vi "Part 1.vi"(11 "Input":string) -> (3 "Output":i64)   [LabVIEW 2021]
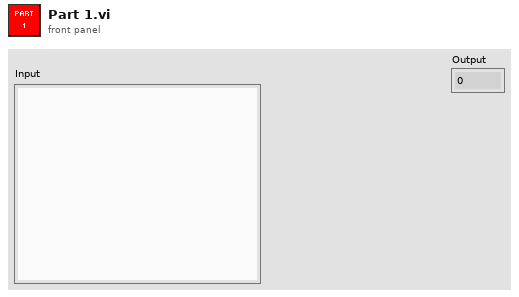
[diagram p1: front panel]
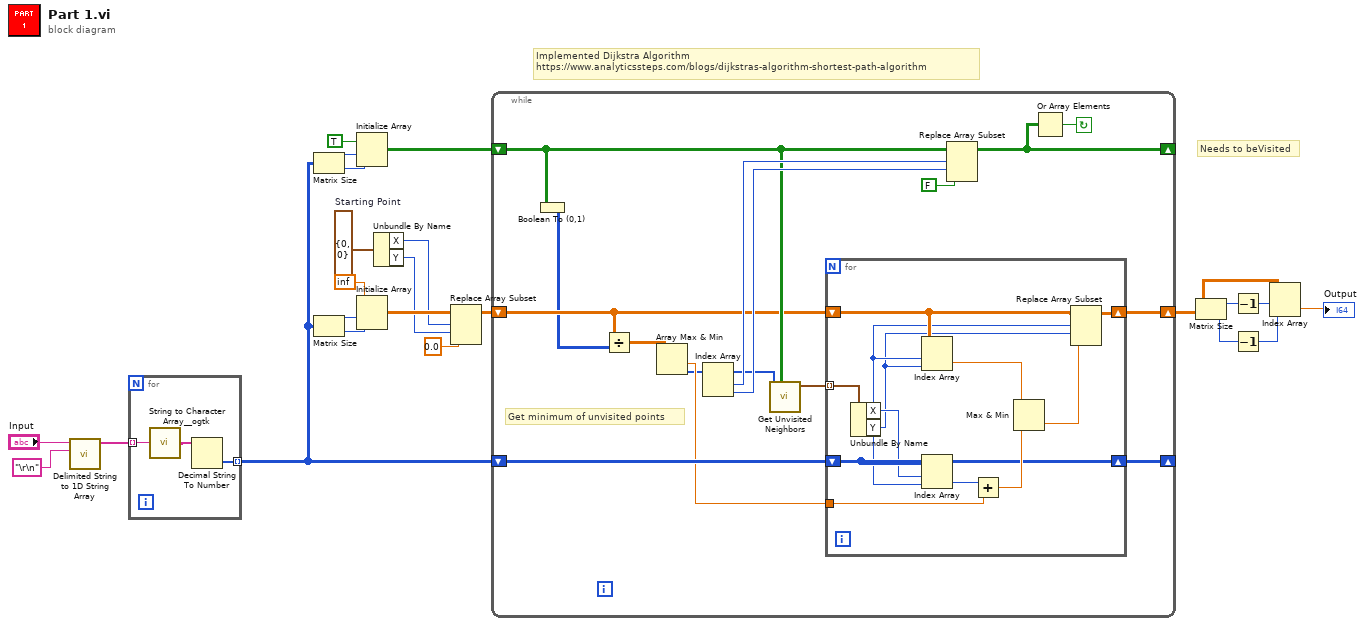
[diagram p0: block diagram]
diagram:
  w9 = cluster{"X":i32, "Y":i32} {"X"=0, "Y"=0}  # Starting Point
  # "Implemented Dijkstra Algorithm\nhttps://www.analyticssteps.com/blogs/dijkstras-algorithm-shortest-path-algorithm"
  # "Needs to beVisited"
  n1 = call <vilib>:"Delimited String to 1D String Array.vi"("delimiter"="\r\n", "delimited string"="Input") -> ("string array"=w21:string[])  [unwired: 9 in]
  n2 = for {
    tunnel: w21 -> [w26] mode=indexing
    tunnel: [w24] -> w12 mode=indexing
    n3 = call <userlib>:"String to Character Array__ogtk.vi"("Input String"=w26) -> ("Character Array"=w25:string[])
    n4 = Decimal String To Number(string=w25) -> (number=w24:i32[])  [unwired: 2 in, 1 out]
  }
  n5 = Matrix Size(0:w12) -> (1:w20:i32, 2:w19:i32)
  n6 = Matrix Size(0:w12) -> (1:w13:i32, 2:w14:i32)
  n7 = Initialize Array(TRUE, w20, w19) -> (w17:bool[][])
  n8 = Initialize Array(inf, w13, w14) -> (w15:dbl[][])
  n9 = Unbundle By Name(w9) -> ("X"=w7:i32, "Y"=w8:i32)
  n10 = Replace Array Subset(array=w15, new element=0.0, index (row)=w7, index (col)=w8) -> (w10:dbl[][])
  n11 = while {
    shift-right: [w39] -> _
    shift-left: w12 -> [w40]
    shift-right: [w34] -> _
    shift-left: w17 -> [w30]
    shift-right: [w37] -> w1
    shift-left: w10 -> [w29]
    stop <- w33 continue-if-true
    # "Get minimum of unvisited points"
    n12 = Boolean To (0,1)(Boolean=w30) -> (0, 1=w28:i16[][])
    n13 = Divide(x=w29, y=w28) -> (x/y=w27:dbl[][])
    n14 = Array Max & Min(array=w27) -> (min value=w38:dbl, min index (indices)=w32:i32[])  [unwired: 2 out]
    n15 = Index Array(array=w32) -> (element #1=w36:i32, element #2=w35:i32)  [unwired: 2 in]
    n16 = call "Get Unvisited Neighbors.vi"("Unvisited"=w30, "Current Point"=w32) -> ("Unvisited Neighbors"=w31:cluster{"X":i32, "Y":i32}[])  [unwired: 9 in]
    n17 = for {
      shift-right: [w46] -> w39
      shift-left: w40 -> [w46]
      tunnel: w38 -> [w52]
      shift-right: [w48] -> w37
      shift-left: w29 -> [w49]
      tunnel: w31 -> [w43] mode=indexing
      n18 = Unbundle By Name(w43) -> ("X"=w45:i32, "Y"=w44:i32)
      n19 = Index Array(array=w49, index (row)=w45, index (col)=w44) -> (element=w50:dbl)
      n20 = Index Array(array=w46, index (row)=w45, index (col)=w44) -> (element=w42:i32)
      n21 = Add(x=w42, y=w52) -> (x+y=w51:dbl)
      n22 = Max & Min(x=w50, y=w51) -> (min(x,y)=w47:dbl)  [unwired: 1 out]
      n23 = Replace Array Subset(array=w49, new element=w47, index (row)=w45, index (col)=w44) -> (w48:dbl[][])
    }
    n24 = Replace Array Subset(array=w30, new element=FALSE, index (row)=w36, index (col)=w35) -> (w34:bool[][])
    n25 = Or Array Elements(Boolean array=w34) -> (logical OR=w33:bool)
  }
  n26 = Matrix Size(0:w1) -> (1:w6:i32, 2:w4:i32)
  n27 = Decrement(x=w6) -> (x-1=w5:i32)
  n28 = Decrement(x=w4) -> (x-1=w3:i32)
  n29 = Index Array(array=w1, index (row)=w5, index (col)=w3) -> (element=→"Output":dbl)
